vi "Init Hardware.vi"(8 "error in (no error)":errorcluster, 11 "Prema Driver in":refnum<class "Prema Driver.lvclass">) -> (0 "error out":errorcluster, 3 "Prema Driver out":refnum<class "Prema Driver.lvclass">)   [LabVIEW 2021, in "Prema Driver.lvclass"]
uses:
  Prema Driver.lvclass
  C:/Git/NHMFL_Core/Libraries/Instruments/Instrument Driver/Instrument Driver.lvclass
  Instrument Driver/Instrument Driver.lvclass/Instrument Driver.ctl
  Instrument Driver/Read Recorder name.vi
  Instrument Driver/Write Channel names.vi
  Instrument Driver/Write Channel units.vi
  Simple VISA Reader/Simple VISA Reader Driver.lvclass
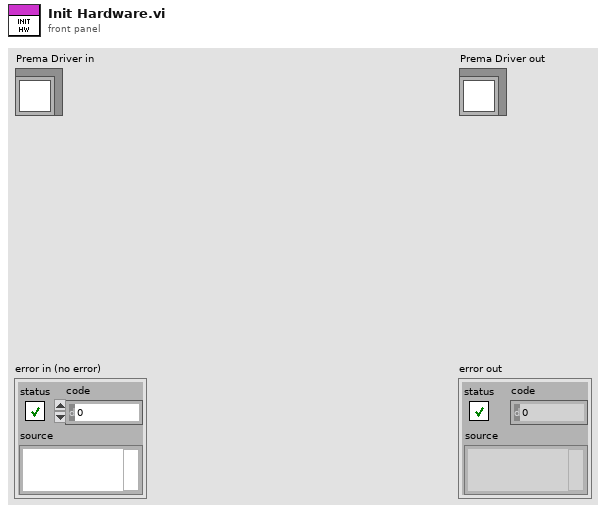
[diagram p1: front panel]
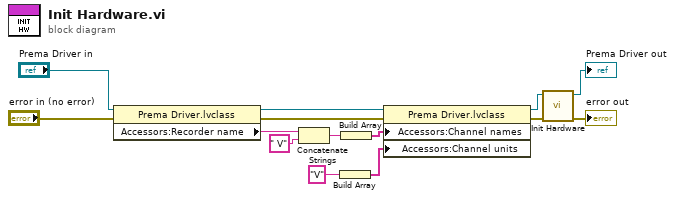
[diagram p0: block diagram]
diagram:
  n1 = property class="Prema Driver.lvclass"(reference="Prema Driver in", error in="error in (no error)") -> (reference out=w12:refnum<class "Prema Driver.lvclass">, error out=w5:errorcluster, "Accessors:Recorder name"=w7:string)
  n2 = Concatenate Strings(w7, " V") -> (w9:string)
  n3 = Build Array("V") -> (w11:string[])
  n4 = Build Array(w9) -> (w6:string[])
  n5 = property class="Prema Driver.lvclass"(reference=w12, error in=w5, "Accessors:Channel names"=w6, "Accessors:Channel units"=w11) -> (reference out=w1:refnum<class "Prema Driver.lvclass">, error out=w3:errorcluster)
  n6 = call-parent "Init Hardware.vi"("error in (no error)"=w3, "Instrument Driver in"=w1) -> ("error out"=→"error out":errorcluster, "Instrument Driver out"=→"Prema Driver out":refnum<class "Prema Driver.lvclass">)  [unwired: 8 in]
